vi "Configure Pre-trigger.vi"(6 "Buffer Control (0: Never)":i32(ring) items=["Never", "Next", "Always", "Pretrigger"], 7 "Pre-trigger Readings Number (0)":dbl, 8 "error in (no error)":errorcluster, 9 "Pre-trigger Readings Percent (50)":dbl=50.0, 10 "Pre-trigger Event (2: Manual)":i32(ring)=2 items=["Trigger Link", "Bus", "Manual"], 11 "VISA resource name":refnum<visa-resource-name>) -> (0 "error out":errorcluster, 3 "VISA resource name out":refnum<visa-resource-name>)   [LabVIEW 2019, in "Keithley 6517.lvlib"]
doc: "Configures pre-trigger readings percent and number, pre-trigger event and buffer control.\n\n<B>Note:</B>\nThis VI is <B>NOT</B> compatible with model <B>6514</B>."
uses:
  Keithley 6517.lvlib
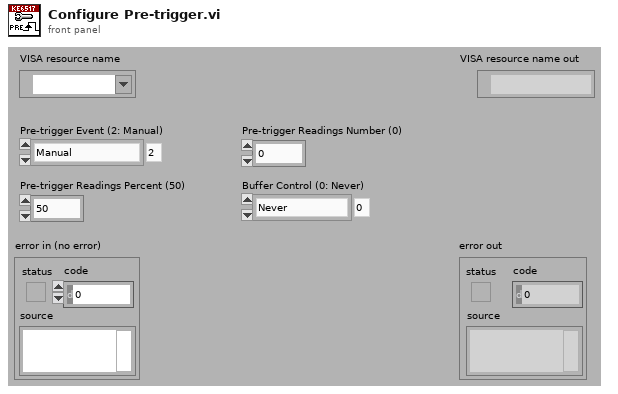
[diagram p1: front panel]
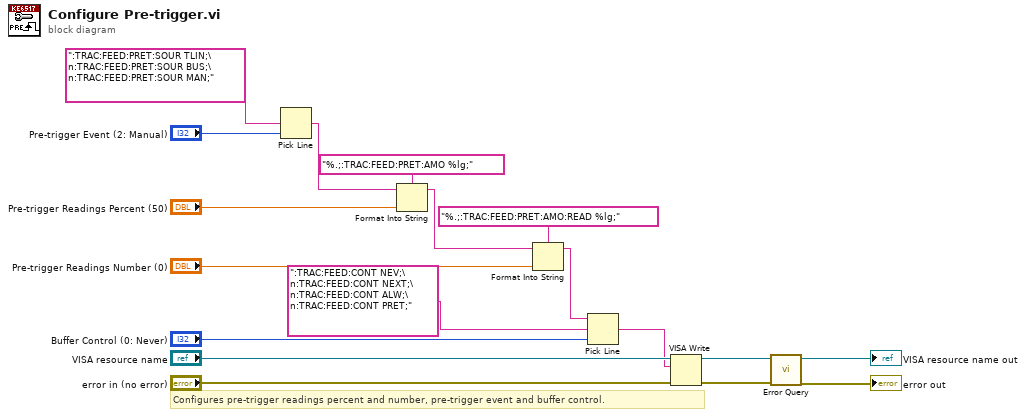
[diagram p0: block diagram]
diagram:
  # "Configures pre-trigger readings percent and number, pre-trigger event and buffer control."
  n1 = Pick Line(multi-line string=":TRAC:FEED:PRET:SOUR TLIN;\n:TRAC:FEED:PRET:SOUR BUS;\n:TRAC:FEED:PRET:SOUR MAN;", line index="Pre-trigger Event (2: Manual)") -> (output string=w2:string)  [unwired: 1 in]
  n2 = Format Into String(format string="%.;:TRAC:FEED:PRET:AMO %lg;", initial string=w2, "Pre-trigger Readings Percent (50)") -> (resulting string=w16:string)  [unwired: 1 in, 1 out]
  n3 = Format Into String(format string="%.;:TRAC:FEED:PRET:AMO:READ %lg;", initial string=w16, "Pre-trigger Readings Number (0)") -> (resulting string=w1:string)  [unwired: 1 in, 1 out]
  n4 = Pick Line(string ("")=w1, multi-line string=":TRAC:FEED:CONT NEV;\n:TRAC:FEED:CONT NEXT;\n:TRAC:FEED:CONT ALW;\n:TRAC:FEED:CONT PRET;", line index="Buffer Control (0: Never)") -> (output string=w3:string)
  n5 = VISA Write(VISA resource name="VISA resource name", write buffer=w3, error in (no error)="error in (no error)") -> (VISA resource name out=w11:refnum<visa-resource-name>, error out=w10:errorcluster)  [unwired: 1 out]
  n6 = call "Error Query.vi"("error in (no error)"=w10, "VISA resource name"=w11) -> ("error out"=→"error out":errorcluster, "VISA resource name out"=→"VISA resource name out":refnum<visa-resource-name>)  [unwired: 6 in, 2 out]
